vi "迭代计算1.vi"() -> ()   [LabVIEW 2014]
uses:
  <vilib>/userdefined/High Color/IMAQdx.ctl
  <vilib>/vision/driver/NI_Vision_Acquisition_Software.lvlib
  <vilib>/vision/NI_Vision_Development_Module.lvlib
panel:
  out "迭代结果":T1(plugin-control)
  out "当前迭代":i32
  out "当前状态":string
  out "x > y?":bool
  in  "迭代次数":u16
  out "序号":i32
  out "输出":T1(plugin-control)
  out "当前图像":string
  in  "分割个数 灰度级":i32=52
  in  "列数":i32=10
  in  "行数":i32=10
  in  "摄像机源":T2
  in  "Stop (F)":bool caption="亮度确认"
  in  "Gain::Value":dbl(slide)=296.0 min=0.0 max=1023.0 step=1.0 scale=0.0..1023.0
  out "当前增益":dbl=296.0 caption="Gain::Value" min=0.0 max=1023.0 step=1.0
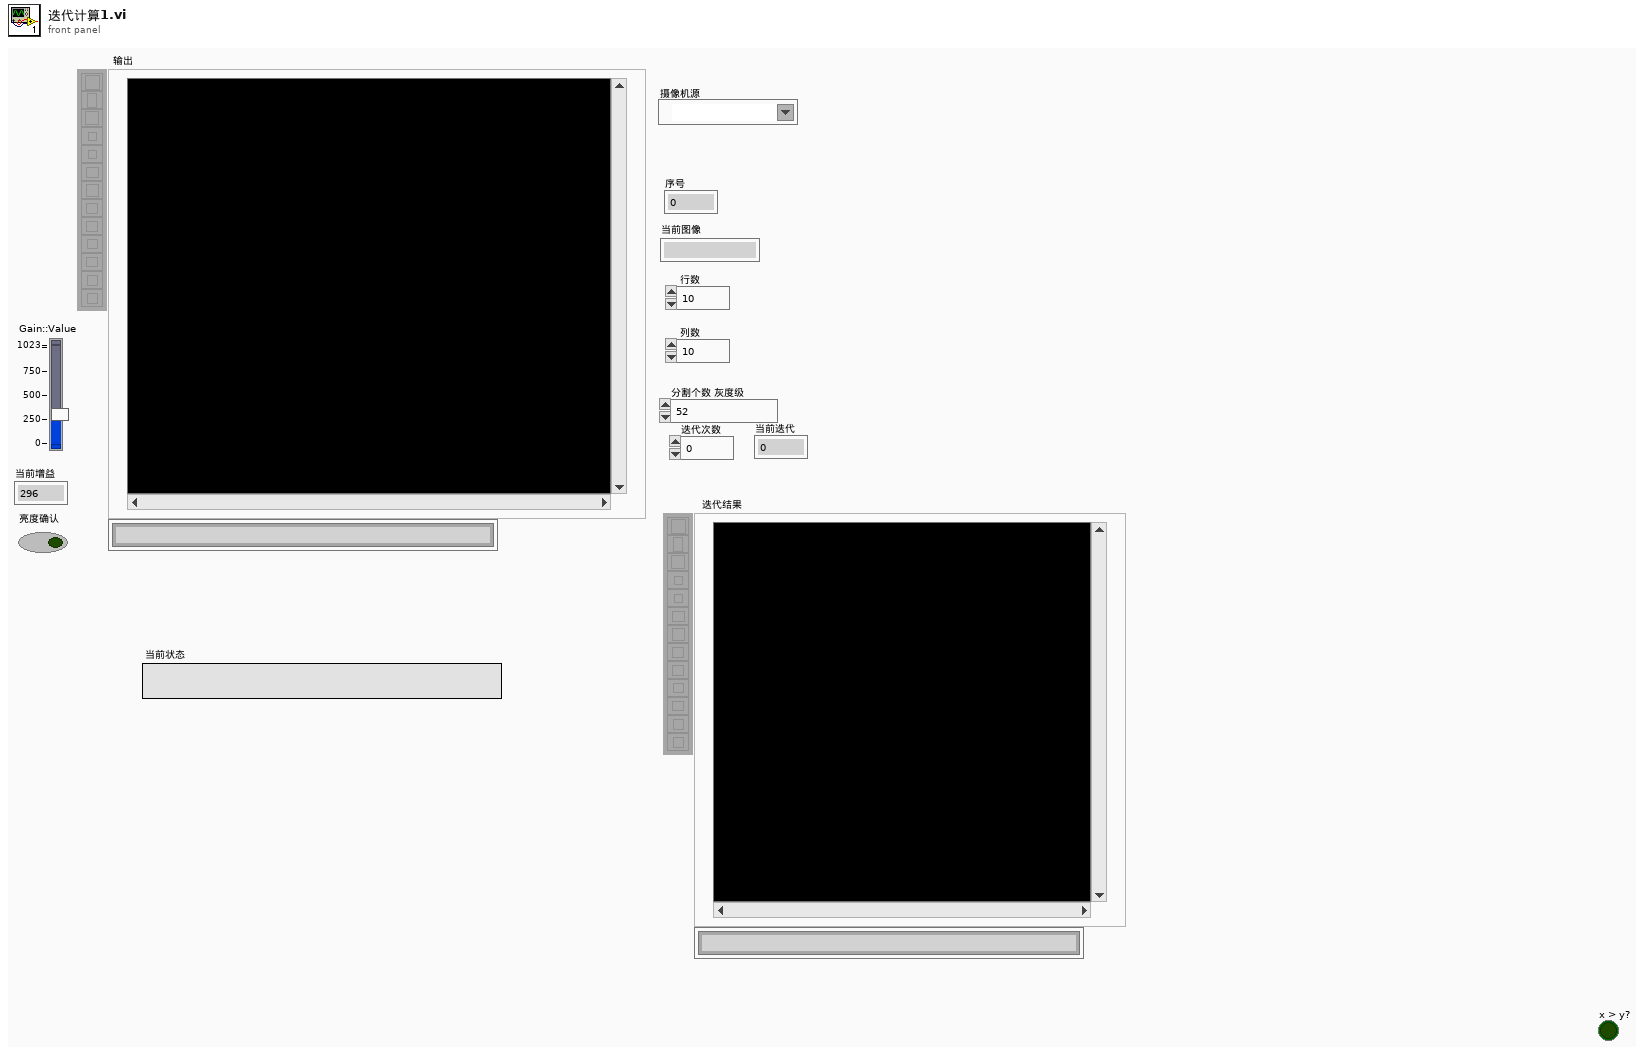
[diagram p1: front panel]
types:
  T1 = typedef "IMAQ Image.ctl" = refnum<image>
  T2 = typedef "IMAQdx.ctl" = refnum<k21>
  T3 = typedef "Image Type" = u32
  T4 = typedef "LVAllMonitorsDisplayTypeDef.ctl" = cluster{"Bounds":cluster{"Left":i16, "Top":i16, "Right":i16, "Bottom":i16}, "Depth":i16}[]
  T5 = typedef "imagedata.ctl" = cluster{"image type":i32, "image depth":i32, "image":u8[], "mask":u8[], "colors":u32[], "Rectangle":cluster{"left":i16, "top":i16, "right":i16, "bottom":i16}}
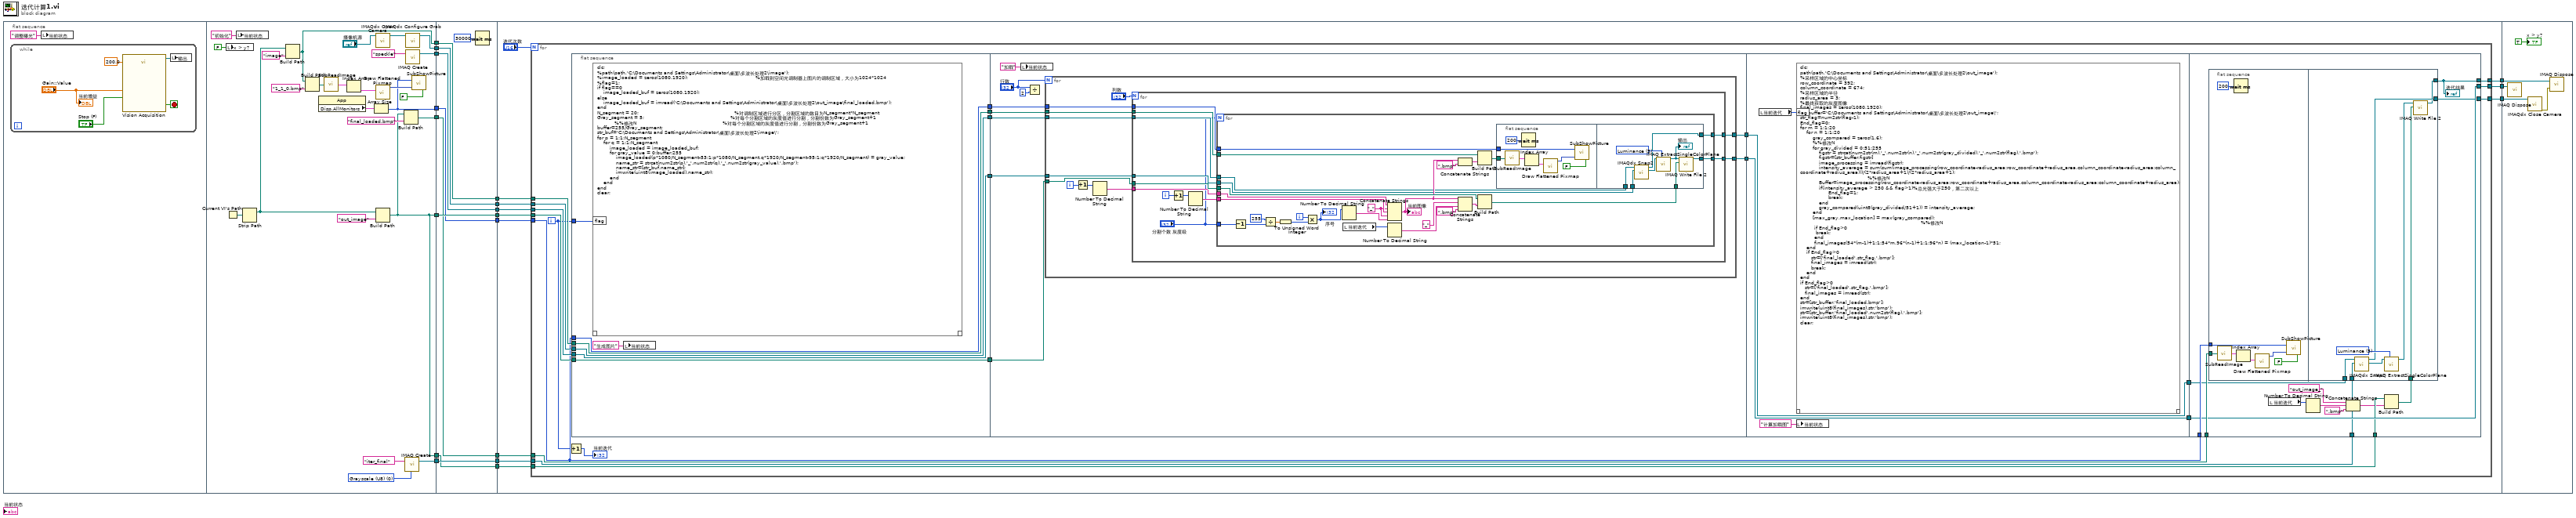
[diagram p0: block diagram]
diagram:
  n1 = flat-sequence {
    tunnel: [w42] -> w19
    tunnel: [w40] -> w18
    tunnel: [w26] -> w17
    tunnel: [w35] -> w16
    tunnel: [w34] -> w15
    tunnel: [w32] -> w6
    tunnel: [w30] -> w4
    tunnel: [w26] -> w1
    tunnel: [w60] -> w14
    tunnel: [w59] -> w13
    tunnel: [w58] -> w12
    tunnel: w19 -> [w58]
    tunnel: w18 -> [w60]
    tunnel: w17 -> [w59]
    tunnel: [w56] -> w11
    tunnel: w16 -> [w56]
    tunnel: [w55] -> w10
    tunnel: w15 -> [w55]
    tunnel: [w54] -> w7
    tunnel: w6 -> [w54]
    tunnel: [w53] -> w5
    tunnel: w4 -> [w53]
    tunnel: [w52] -> w2
    tunnel: w1 -> [w52]
    tunnel: w14 -> [w72]
    tunnel: w13 -> [w71]
    tunnel: w12 -> [w70]
    tunnel: w11 -> [w69]
    tunnel: w10 -> [w68]
    tunnel: [w67] -> w9
    tunnel: [w66] -> w8
    tunnel: w7 -> [w64]
    tunnel: w5 -> [w63]
    tunnel: [w62] -> w3
    tunnel: w2 -> [w61]
    tunnel: w9 -> [w214]
    tunnel: w8 -> [w213]
    tunnel: w3 -> [w212]
    frame #0 {
      n2 = while {
        stop <- w24 stop-if-true
        n3 = call "Vision Acquisition"("Gain::Value"="Gain::Value", "Shutter::Value"=200.0, "Stop (F)"="Stop (F)") -> ("Image Out"=w22:T1, "Stopped"=w24:bool)  [unwired: 22 in, 1 out]
        n4 = local write "输出"(w22) -> ()
        "当前增益" <- "Gain::Value"
      }
      n5 = local write "当前状态"("调整曝光" ("当前状态")) -> ()
    }
    frame #1 {
      w29 = T3 0 items=["Grayscale (U8)", "Grayscale (I16)", "Grayscale (SGL)", "Complex (CSG)", "RGB (U32)", "HSL (U32)", "RGB (U64)", "Grayscale (U16)"] ("Image Type")
      n6 = Current VI's Path() -> (path=w50:path)
      n7 = local write "x > y?"(FALSE) -> ()
      n8 = local write "当前状态"("初始化" ("当前状态")) -> ()
      n9 = Strip Path(path=w50) -> (stripped path=w49:path)  [unwired: 1 out]
      n10 = Build Path(base path=w49, name or relative path="image" ("名称或相对路径")) -> (appended path=w40:path)
      n11 = Build Path(base path=w40, name or relative path="1_1_0.bmp" ("名称或相对路径")) -> (appended path=w39:path)
      n12 = property class="App"() -> ("Disp.AllMonitors"=w47:T4)  [unwired: 2 in, 2 out]
      n13 = call "SubReadImage.vi"("Path"=w39) -> ("Image Array"=w46:T5[])  [unwired: 3 in, 1 out]
      n14 = Index Array(array=w46) -> (element=w45:T5)  [unwired: 1 in]
      n15 = Array Size(array=w47) -> (size(s)=w42:i32)
      n16 = call <vilib>:"Draw Flattened Pixmap.vi"("image data"=w45) -> ("new picture"=w44:picture)  [unwired: 8 in]
      n17 = call <vilib>:"IMAQdx Open Camera.vi"("Session In"="摄像机源") -> ("Session Out"=w36:T2)  [unwired: 9 in, 1 out]
      n18 = Build Path(base path=w49, name or relative path="out_image" ("名称或相对路径")) -> (appended path=w26:path)
      n19 = Build Path(base path=w26, name or relative path="final_loaded.bmp" ("名称或相对路径")) -> (appended path=w30:path)
      n20 = call "IMAQ Create"("Image Name"="iter_final", "Image Type"=w29) -> ("New Image"=w32:T1)  [unwired: 3 in, 1 out]
      n21 = call <vilib>:"IMAQdx Configure Grab.vi"("Session In"=w36) -> ("Session Out"=w34:T2)  [unwired: 9 in, 1 out]
      n22 = call "IMAQ Create"("Image Name"="speckle") -> ("New Image"=w35:T1)  [unwired: 4 in, 1 out]
      n23 = call "SubShowPicture.vi"("End"=FALSE, "Picture"=w44, "number of displays"=w42) -> ()  [unwired: 1 in]
    }
    frame #2 {
      n24 = Wait (ms)(milliseconds to wait=u32 30000 ("等待时间（毫秒）")) -> ()  [unwired: 1 out]
    }
    frame #3 {
      n25 = for {
        N: "迭代次数" -> [_]
        tunnel: w72 -> [w94]
        tunnel: w71 -> [w93]
        tunnel: w70 -> [w76]
        tunnel: w69 -> [w92]
        tunnel: [w90] -> w66
        tunnel: w68 -> [w91]
        tunnel: [w75] -> w67
        tunnel: w64 -> [w78]
        tunnel: w63 -> [w77]
        tunnel: [w79] -> w62
        tunnel: w61 -> [w74]
        i -> [w73]
        n26 = Increment(x=w73) -> (x+1=→"当前迭代":i32)
        n27 = flat-sequence {
          tunnel: w91 -> [w97]
          tunnel: w92 -> [w98]
          tunnel: w76 -> [w99]
          tunnel: w93 -> [w100]
          tunnel: w94 -> [w101]
          tunnel: [w101] -> w87
          tunnel: [w100] -> w86
          tunnel: [w99] -> w85
          tunnel: [w98] -> w84
          tunnel: [w97] -> w83
          tunnel: w73 -> [w95]
          tunnel: [w106] -> w89
          tunnel: [w105] -> w88
          tunnel: w87 -> [w111]
          tunnel: w86 -> [w110]
          tunnel: w85 -> [w109]
          tunnel: w84 -> [w108]
          tunnel: w83 -> [w107]
          tunnel: w89 -> [w181]
          tunnel: w88 -> [w180]
          tunnel: [w181] -> w81
          tunnel: [w180] -> w80
          tunnel: [w192] -> w90
          tunnel: w81 -> [w193]
          tunnel: w80 -> [w192]
          tunnel: [w189] -> w79
          tunnel: w78 -> [w190]
          tunnel: w77 -> [w195]
          tunnel: w76 -> [w194]
          tunnel: [w191] -> w75
          tunnel: w74 -> [w188]
          frame #0 {
            n28 = script code="clc;\n%path(path,'C:\\Documents and Settings\\Administrator\\桌面\\多波长处理2\\image');\n%image_loaded = zeros(1080,1920);                                           %加载到空间光调制器上图片的调制区域，大小为1024*1024\n%flag=1;\nif flag==0\n    image_loaded_buf = zeros(1080,1920); \nelse\n    image_loaded_buf = imread('C:\\Documents and Settings\\Administrator\\桌面\\多波长处理2\\out_image\\final_loaded.bmp'); \nend\nN_segment = 20;                                                             %对调制区域进行分区，分割区域的数目为N_segment*N_segment\nGray_segment = 5;                                                       %对每个分割区域的灰度值进行分割，分割份数为Gray_segment+1\n           %%修改N                                                       %对每个分割区域的灰度值进行分割，分割份数为Gray_segment+1\nbuffer=255/Gray_segment;\nstr_buf='C:\\Documents and Settings\\Administrator\\桌面\\多波长处理2\\image\\';\nfor p = 1:1:N_segment\n    for q = 1:1:N_segment\n        image_loaded = image_loaded_buf;\n        for gray_value = 0:buffer:255\n            image_loaded(p*1080/N_segment-53:1:p*1080/N_segment,q*1920/N_segment-95:1:q*1920/N_segment) = gray_value;\n            name_str = strcat(num2str(p),'_',num2str(q),'_',num2str(gray_value),'.bmp');\n            name_str=[str_buf,name_str];\n            imwrite(uint8(image_loaded),name_str);\n        end\n    end\nend\nclear;"("flag"=w95) -> ()  [unwired: 1 in, 1 out]
            n29 = local write "当前状态"("生成图片" ("当前状态")) -> ()
          }
          frame #1 {
            n30 = local write "当前状态"("加载" ("当前状态")) -> ()
            n31 = Divide(x="行数", y=2) -> ()  [unwired: 1 out]
            n32 = for {
              N: "行数" -> [_]
              tunnel: w111 -> [w122]
              tunnel: w110 -> [w121]
              tunnel: w109 -> [w120]
              tunnel: w108 -> [w115]
              tunnel: w107 -> [w114]
              tunnel: [w113] -> w106
              tunnel: [w112] -> w105
              i -> [w118]
              n33 = Increment(x=w118) -> (x+1=w117:i32)
              n34 = Number To Decimal String(number=w117) -> (decimal integer string=w116:string)  [unwired: 1 in]
              n35 = for {
                N: "列数" -> [_]
                tunnel: w122 -> [w134]
                tunnel: w121 -> [w133]
                tunnel: w120 -> [w132]
                tunnel: w116 -> [w128]
                tunnel: w115 -> [w127]
                tunnel: w114 -> [w126]
                tunnel: [w125] -> w113
                tunnel: [w124] -> w112
                i -> [w131]
                n36 = Increment(x=w131) -> (x+1=w130:i32)
                n37 = Number To Decimal String(number=w130) -> (decimal integer string=w129:string)  [unwired: 1 in]
                n38 = for {
                  N: "分割个数 灰度级" -> [_]
                  tunnel: w134 -> [w159]
                  tunnel: w133 -> [w160]
                  tunnel: w132 -> [w157]
                  tunnel: w129 -> [w154]
                  tunnel: w128 -> [w152]
                  tunnel: w127 -> [w148]
                  tunnel: w126 -> [w147]
                  tunnel: [w146] -> w125
                  tunnel: [w144] -> w124
                  tunnel: "分割个数 灰度级" -> [w142]
                  i -> [w156]
                  w153 = "_" ("字符串")
                  n39 = Decrement(x=w142) -> (x-1=w141:i32)
                  n40 = Divide(x=255, y=w141) -> (x/y=w139:dbl)
                  n41 = To Unsigned Word Integer(number=w139) -> (unsigned 16bit integer=w140:u16)
                  n42 = Multiply(x=w156, y=w140) -> (x*y=w155:i32)
                  "序号" <- w155
                  n43 = Number To Decimal String(number=w155) -> (decimal integer string=w161:string)  [unwired: 1 in]
                  n44 = local read "当前迭代"() -> (w138:i32)
                  n45 = Concatenate Strings(w152, w153, w154, w153, w161) -> (w149:string)
                  "当前图像" <- w149
                  n46 = Number To Decimal String(number=w138) -> (decimal integer string=w136:string)  [unwired: 1 in]
                  n47 = Concatenate Strings(w149, ".bmp") -> (w151:string)
                  n48 = Concatenate Strings(w149, "_" ("字符串"), w136, ".bmp" ("字符串")) -> (w162:string)
                  n49 = Build Path(base path=w159, name or relative path=w151) -> (appended path=w158:path)
                  n50 = Build Path(base path=w160, name or relative path=w162) -> (appended path=w145:path)
                  n51 = flat-sequence {
                    tunnel: w158 -> [w169]
                    tunnel: w157 -> [w165]
                    tunnel: w148 -> [w176]
                    tunnel: w147 -> [w175]
                    tunnel: [w174] -> w146
                    tunnel: w145 -> [w172]
                    tunnel: [w171] -> w144
                    frame #0 {
                      n52 = call "SubReadImage.vi"("Path"=w169) -> ("Image Array"=w168:T5[])  [unwired: 3 in, 1 out]
                      n53 = Wait (ms)(milliseconds to wait=200) -> ()  [unwired: 1 out]
                      n54 = Index Array(array=w168) -> (element=w167:T5)  [unwired: 1 in]
                      n55 = call <vilib>:"Draw Flattened Pixmap.vi"("image data"=w167) -> ("new picture"=w166:picture)  [unwired: 8 in]
                      n56 = call "SubShowPicture.vi"("End"=FALSE, "Picture"=w166, "number of displays"=w165) -> ()  [unwired: 1 in]
                    }
                    frame #1 {
                      w177 = 5 items=["Red", "Green", "Blue", "Hue", "Saturation", "Luminance", "Value", "Intensity"] ("Color Plane")
                      n57 = call <vilib>:"IMAQdx Snap2.vi"("Image In"=w176, "Session In"=w175) -> ("Image Out"=w170:T1, "Session Out"=w174:T2)  [unwired: 7 in, 1 out]
                      n58 = call "IMAQ ExtractSingleColorPlane"("Color Plane"=w177, "Image Src"=w170) -> ("Image Dst Out"=w173:T1)  [unwired: 8 in, 1 out]
                      "输出" <- w173
                      n59 = call-poly "IMAQ Write File 2"("File Path"=w172, "Image"=w173) -> ("Image Out (duplicate)"=w171:T1)  [unwired: 8 in, 1 out]
                    }
                  }
                }
              }
            }
          }
          frame #2 {
            n60 = local read "当前迭代"() -> (w178:i32)
            n61 = script code="clc;\npath(path,'C:\\Documents and Settings\\Administrator\\桌面\\多波长处理2\\out_image');\n%采样区域的中心坐标\nrow_coordinate = 392;\ncolumn_coordinate = 674;\n%采样区域的半径\nradius_area = 3;\n%最终获取的灰度图像\nfinal_images = zeros(1080,1920);\nstr_buffer='C:\\Documents and Settings\\Administrator\\桌面\\多波长处理2\\out_image\\';\nstr_flag=num2str(flag-1);\nEnd_flag=0;\nfor m = 1:1:20\n    for n = 1:1:20\n        gray_compared = zeros(1,6);\n        %%修改N\n        for gray_divided = 0:51:255\n            figstr = strcat(num2str(m),'_',num2str(n),'_',num2str(gray_divided),'_',num2str(flag),'.bmp');\n            figstr=[str_buffer,figstr]\n            image_processing = imread(figstr);\n            intensity_average = sum(sum(image_processing(row_coordinate-radius_area:row_coordinate+radius_area,column_coordinate-radius_area:column_coordinate+radius_area)))/(2*radius_area+1)/(2*radius_area+1);\n                                           %%修改N\n            Buffer=image_processing(row_coordinate-radius_area:row_coordinate+radius_area,column_coordinate-radius_area:column_coordinate+radius_area);\n            if(intensity_average > 250 && flag>1)%总光强大于250，第二次以上\n                  End_flag=1;\n                  break;\n            end\n            gray_compared(uint8(gray_divided/51+1)) = intensity_average;\n        end\n        [max_gray,max_location] = max(gray_compared);\n                                                                             %%修改N\n         if End_flag>0\n          break;\n         end\n         final_images(54*(m-1)+1:1:54*m,96*(n-1)+1:1:96*n) = (max_location-1)*51;\n    end\n    if End_flag>0\n       str=['final_loaded',str_flag,'.bmp'];\n       final_images = imread(str);\n       break;\n    end\nend\nif End_flag>0\n   str=['final_loaded',str_flag,'.bmp'];\n   final_images = imread(str);\nend\nstr=[str_buffer,'final_loaded.bmp'];\nimwrite(uint8(final_images),str,'bmp'); \nstr=[str_buffer,'final_loaded',num2str(flag),'.bmp'];\nimwrite(uint8(final_images),str,'bmp'); \nclear;"("flag"=w178) -> ()  [unwired: 1 in, 1 out]
            n62 = local write "当前状态"("计算加载图" ("当前状态")) -> ()
          }
          frame #3 {
            n63 = flat-sequence {
              tunnel: w195 -> [w198]
              tunnel: w194 -> [w197]
              tunnel: w193 -> [w209]
              tunnel: [w208] -> w191
              tunnel: w190 -> [w207]
              tunnel: [w204] -> w189
              tunnel: w183 -> [w206]
              frame #0 {
                n64 = call "SubReadImage.vi"("Path"=w198) -> ("Image Array"=w202:T5[])  [unwired: 3 in, 1 out]
                n65 = Wait (ms)(milliseconds to wait=200) -> ()  [unwired: 1 out]
                n66 = Index Array(array=w202) -> (element=w201:T5)  [unwired: 1 in]
                n67 = call <vilib>:"Draw Flattened Pixmap.vi"("image data"=w201) -> ("new picture"=w200:picture)  [unwired: 8 in]
                n68 = call "SubShowPicture.vi"("End"=FALSE, "Picture"=w200, "number of displays"=w197) -> ()  [unwired: 1 in]
              }
              frame #1 {
                w210 = 5 items=["Red", "Green", "Blue", "Hue", "Saturation", "Luminance", "Value", "Intensity"] ("Color Plane")
                n69 = call <vilib>:"IMAQdx Snap2.vi"("Image In"=w207, "Session In"=w209) -> ("Image Out"=w203:T1, "Session Out"=w208:T2)  [unwired: 7 in, 1 out]
                n70 = call "IMAQ ExtractSingleColorPlane"("Color Plane"=w210, "Image Src"=w203) -> ("Image Dst Out"=w205:T1)  [unwired: 8 in, 1 out]
                n71 = call-poly "IMAQ Write File 2"("File Path"=w206, "Image"=w205) -> ("Image Out (duplicate)"=w204:T1)  [unwired: 8 in, 1 out]
              }
            }
            n72 = local read "当前迭代"() -> (w182:i32)
            n73 = Number To Decimal String(number=w182) -> (decimal integer string=w186:string)  [unwired: 1 in]
            n74 = Concatenate Strings("out_image_" ("名称或相对路径"), w186, ".bmp") -> (w184:string)
            n75 = Build Path(base path=w188, name or relative path=w184) -> (appended path=w183:path)
            "迭代结果" <- w189
          }
        }
      }
    }
    frame #4 {
      n76 = call "IMAQ Dispose"("Image"=w213) -> ()  [unwired: 5 in, 1 out]
      n77 = call <vilib>:"IMAQdx Close Camera.vi"("Session In"=w214) -> ("error out"=w211:errorcluster)  [unwired: 10 in]
      n78 = call "IMAQ Dispose"("Image"=w212, "error in (no error)"=w211) -> ()  [unwired: 4 in, 1 out]
      "x > y?" <- TRUE
    }
  }
